vi "周期启动 (子VI).vi"   [LabVIEW 2016, in "质控单元.lvlib"]
types:
  T1 = cluster{"是否启用仪器":bool, "CODMn":cluster{"启动测量模式":cluster{"测量模式":enum16{"水样测量", "标样核查", "加标回收", "平行样", "校零", "校标"}}, "确定按钮":bool}, "启动模块":cluster{"氨氮":bool, "总磷":bool, "总氮":bool, "CODMn":bool, "CODCr":bool}, "常规启动":bool, "直接启动":bool}
  T2 = cluster{"周期设置类型":enum16{"定点启动", "间隔启动"}, "定时功能启用":bool, "定时间隔":dbl, "间隔启动次数 ":dbl, "已经启动次数 ":dbl, "24H周期设置":bool[], "模块选择":cluster{"氨氮":bool, "总磷":bool, "总氮":bool, "CODMn":bool, "CODCr":bool}, "采配水启用":bool}
  T3 = typedef "LVDateTimeRec.ctl" = cluster{"秒数的小数部分":dbl, "秒":i32, "分":i32, "时":i32, "日":i32, "月":i32, "年":i32, "天数（周）":i32, "天数（年）":i32, "DST":i32}
  T4 = cluster{"氨氮":bool, "总磷":bool, "总氮":bool, "CODMn":bool, "CODCr":bool}
  T5 = enum32{"Bad", "Idle", "Run top level", "Running"}
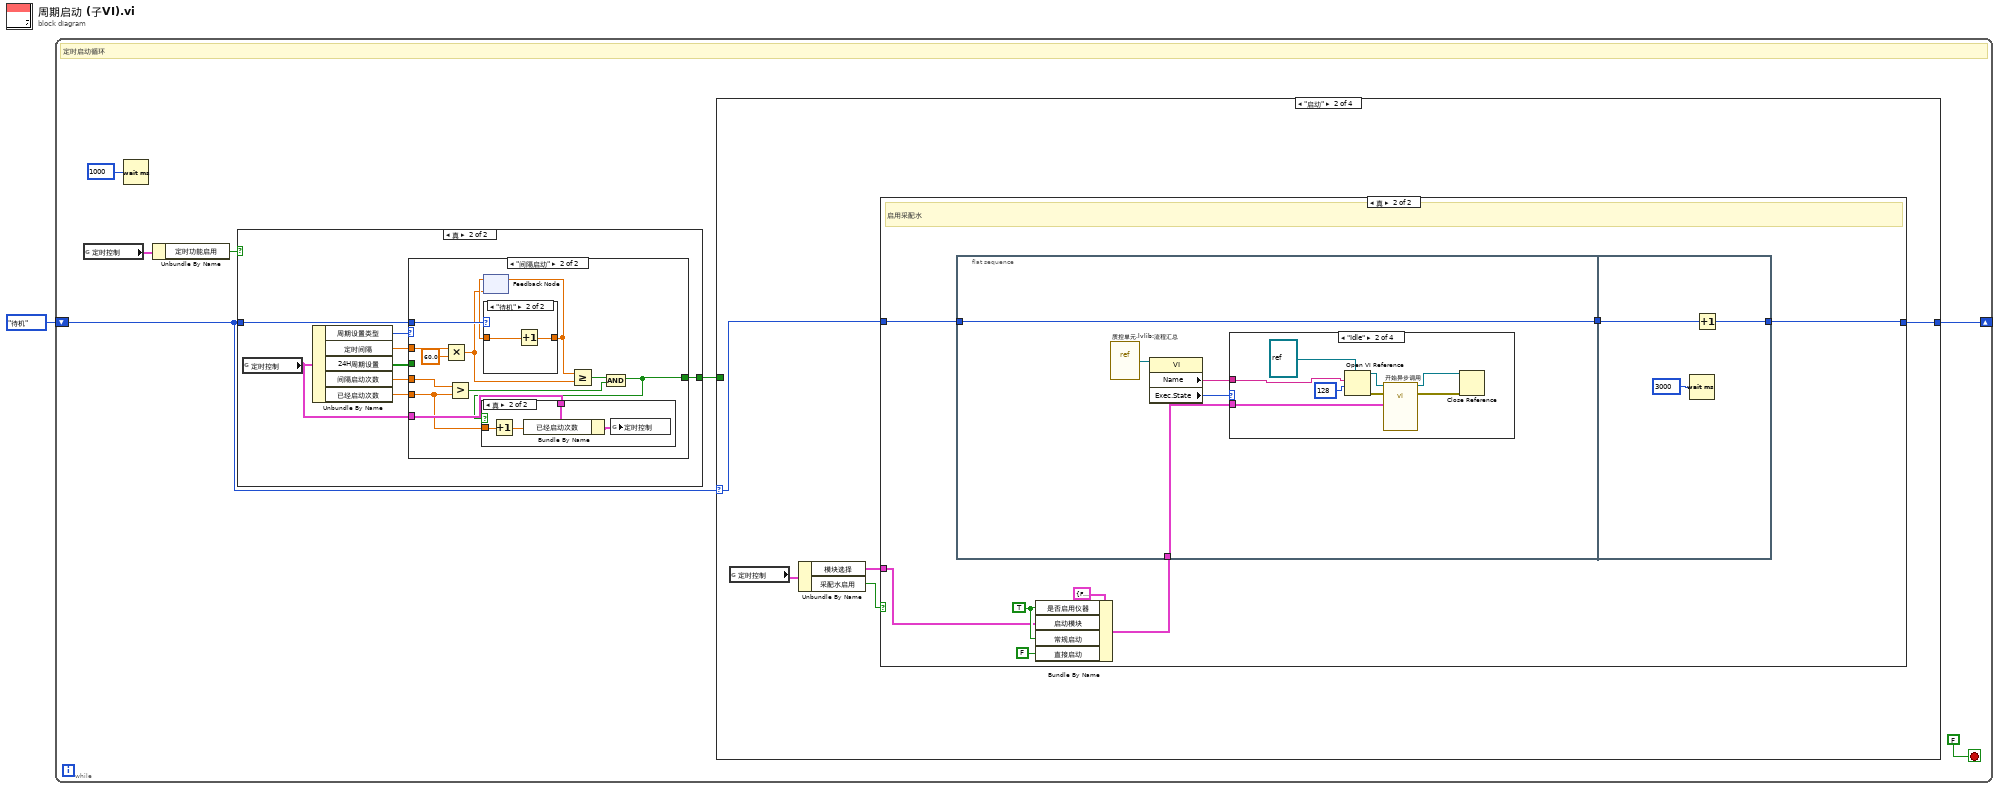
[diagram p0: block diagram]
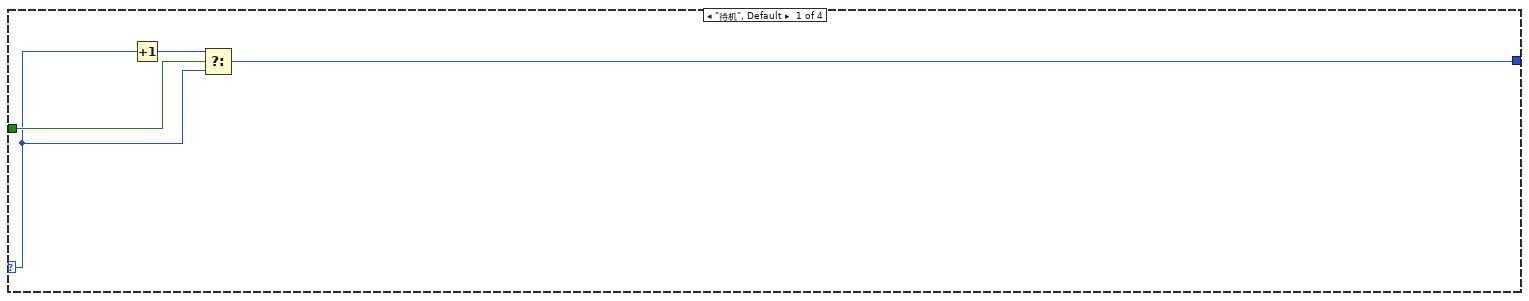
[diagram p2: hidden frame]
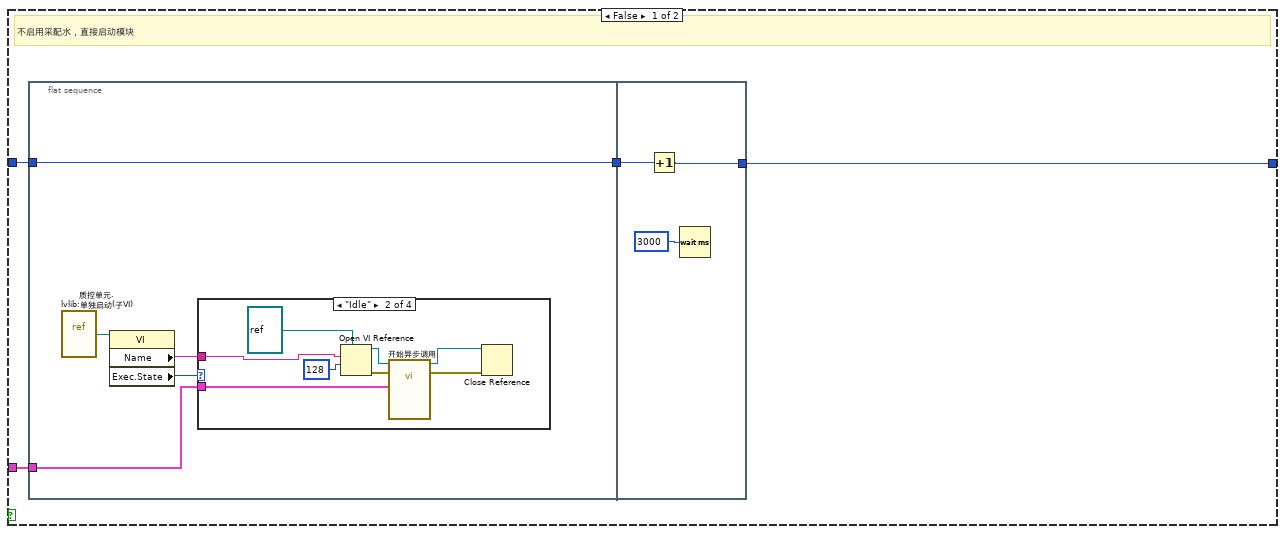
[diagram p3: hidden frame]
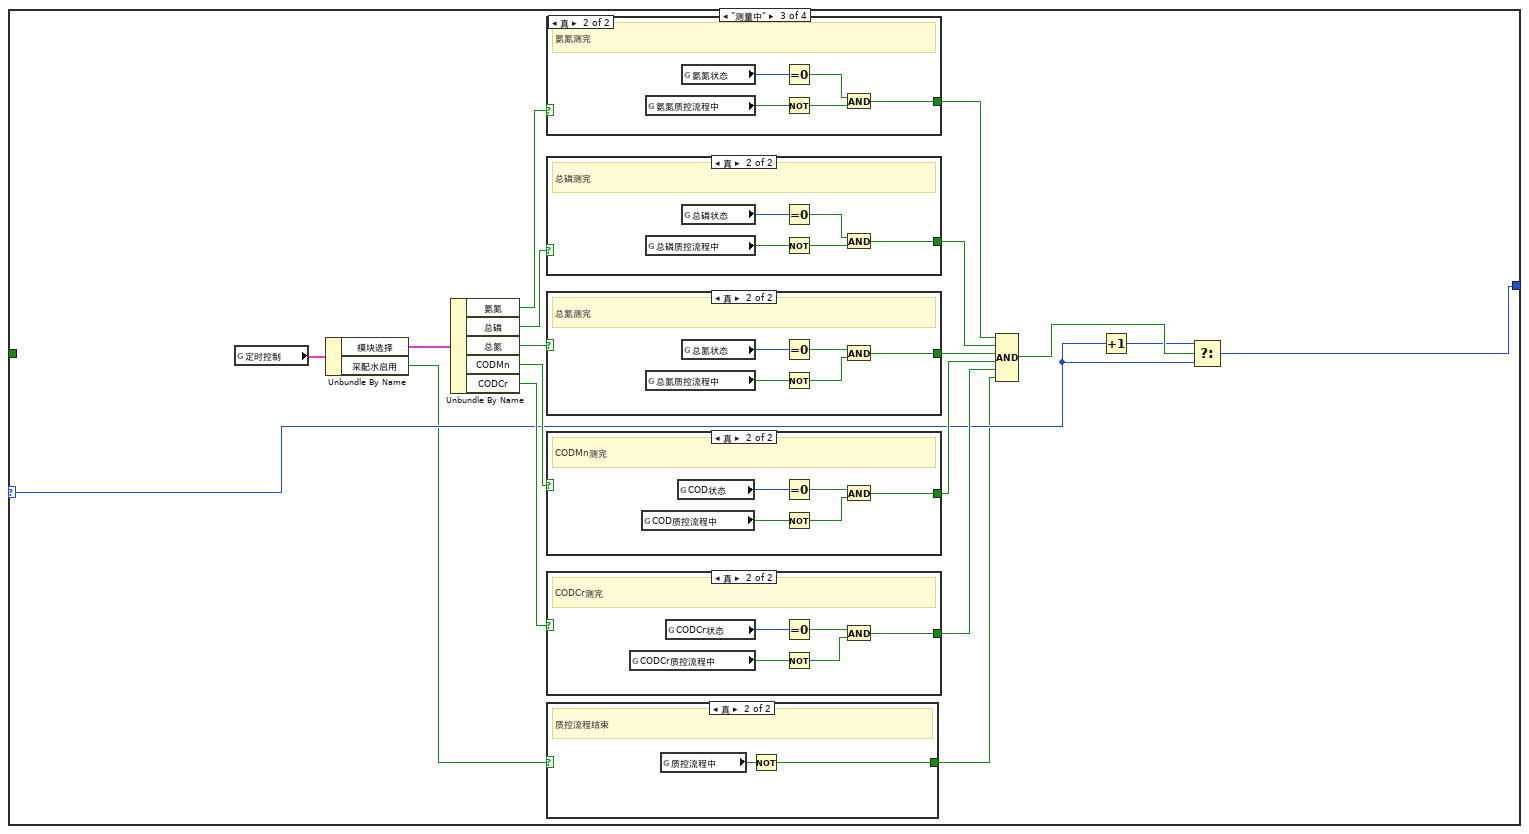
[diagram p10: hidden frame]
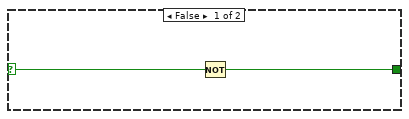
[diagram p11: hidden frame]
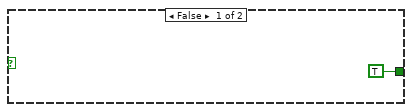
[diagram p12: hidden frame]
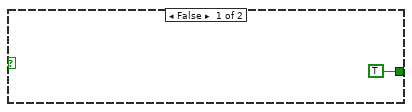
[diagram p13: hidden frame]
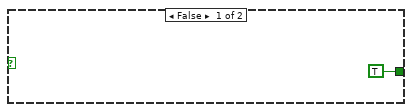
[diagram p14: hidden frame]
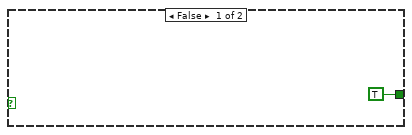
[diagram p15: hidden frame]
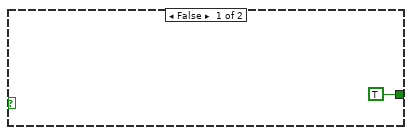
[diagram p16: hidden frame]
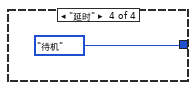
[diagram p17: hidden frame]
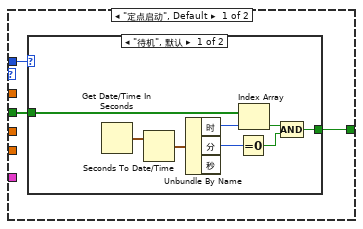
[diagram p19: hidden frame]
diagram:
  n1 = while {
    shift-right: [w6] -> _
    shift-left: enum16{"待机", "启动", "测量中", "延时"}."待机" -> [w5]
    stop <- FALSE stop-if-true
    # "定时启动循环"
    n2 = global read "断电保存全局.vi" "定时控制"() -> (w3:T2)
    n3 = Wait (ms)(milliseconds to wait=u32 1000 ("等待时间（毫秒）")) -> ()  [unwired: 1 out]
    n4 = Unbundle By Name(w3) -> ("定时功能启用"=w2:bool)
    n5 = case shown="真" w2 {
      tunnel: w5 -> [_ w119]
      tunnel: [_ w118] -> w4
      frame False {
      }
      frame True {
        n6 = global read "断电保存全局.vi" "定时控制"() -> (w115:T2)
        n7 = Unbundle By Name(w115) -> ("周期设置类型"=w120:enum16{"定点启动", "间隔启动"}, "定时间隔"=w121:dbl, "24H周期设置"=w122:bool[], "间隔启动次数"=w117:dbl, "已经启动次数"=w116:dbl)
        n8 = case shown="\"间隔启动\"" w120 {
          tunnel: w121 -> [_ w142]
          tunnel: w122 -> [w125 _]
          tunnel: w119 -> [w123 w145]
          tunnel: [w124 w134] -> w118
          tunnel: w117 -> [_ w138]
          tunnel: w116 -> [_ w135]
          tunnel: w115 -> [_ w136]
          frame "定点启动", Default {
            n9 = case shown="\"待机\", 默认" w123 {
              tunnel: w125 -> [w131 _]
              tunnel: [w126 _] -> w124
              frame "待机", Default {
                n10 = Get Date/Time In Seconds() -> (seconds since 1Jan1904=w133:timestamp)
                n11 = Seconds To Date/Time(time stamp (now)=w133) -> (date time rec=w132:T3)  [unwired: 1 in]
                n12 = Unbundle By Name(w132) -> ("时"=w130:i32, "分"=w129:i32)  [unwired: 1 out]
                n13 = Equal To 0?(x=w129) -> (x = 0?=w127:bool)
                n14 = Index Array(array=w131, index=w130) -> (element=w128:bool)
                n15 = Compound Arithmetic op=AND ("复合运算")(w128, w127) -> (w126:bool)
              }
              frame "启动" {
              }
            }
          }
          frame "间隔启动" {
            n16 = Multiply(x=w142, y=60.0) -> (x*y=w139:dbl)
            n17 = Greater?(x=w138, y=w135) -> (0:w137:bool)
            n18 = feedback #1(w139) -> (w144:dbl)
            n19 = case shown="\"待机\"" w145 {
              tunnel: w144 -> [_ w151]
              tunnel: [_ w150] -> w143
              frame Default {
              }
              frame "待机" {
                n20 = Increment(x=w151) -> (x+1=w150:dbl)
              }
            }
            n21 = feedback-in #1(w143) -> ()
            n22 = Greater Or Equal?(x=w143, y=w139) -> (x >= y?=w140:bool)
            n23 = And(x=w140, y=w137) -> (x .and. y?=w134:bool)
            n24 = case shown="真" w134 {
              tunnel: w136 -> [_ w149]
              tunnel: w135 -> [_ w148]
              frame False {
              }
              frame True {
                n25 = Increment(x=w148) -> (x+1=w147:dbl)
                n26 = Bundle By Name(cluster=w149, "已经启动次数"=w147) -> (w146:T2)
                n27 = global write "断电保存全局.vi" "定时控制"(w146) -> ()
              }
            }
          }
        }
      }
    }
    n28 = case shown="\"启动\"" w5 {
      selector: w5 -> [w9 w14 w65 _]
      tunnel: [w11 w17 w66 enum16{"待机", "启动", "测量中", "延时"}."待机"] -> w6
      tunnel: w4 -> [w12 _ _ _]
      frame "待机", Default {
        n29 = Increment(x=w9) -> (x+1=w10:enum16{"待机", "启动", "测量中", "延时"})
        n30 = Select(t=w10, s=w12, f=w9) -> (s? t:f=w11:enum16{"待机", "启动", "测量中", "延时"})
      }
      frame "启动" {
        n31 = global read "断电保存全局.vi" "定时控制"() -> (w15:T2)
        n32 = Unbundle By Name(w15) -> ("模块选择"=w16:T4, "采配水启用"=w13:bool)
        n33 = case shown="真" w13 {
          tunnel: [w20 w43] -> w17
          tunnel: w16 -> [w19 w39]
          tunnel: w14 -> [w18 w44]
          frame False {
            # "不启用采配水，直接启动模块"
            n34 = flat-sequence {
              tunnel: w19 -> [w22]
              tunnel: w18 -> [w26]
              tunnel: [w26] -> w21
              tunnel: [w37] -> w20
              tunnel: w21 -> [w36]
              frame #0 {
                n35 = vi-ref "质控单元.lvlib:单独启动(子VI).vi"() -> (w24:refnum<vi>)
                n36 = property class="VI"(reference=w24) -> ("Name"=w25:string, "Exec.State"=w23:T5)  [unwired: 1 in, 2 out]
                n37 = case shown="\"Idle\"" w23 {
                  tunnel: w25 -> [_ w33 _ _]
                  tunnel: w22 -> [_ w27 _ _]
                  frame "Bad", Default {
                  }
                  frame "Idle" {
                    n38 = Open VI Reference(type specifier VI Refnum (for type only)=refnum<vi> refnum ("类型说明符VI引用句柄（仅用于类型）"), vi path=w33, options=128 ("选项")) -> (vi reference=w34:refnum<vi>, error out=w30:errorcluster)  [unwired: 3 in]
                    n39 = call-by-ref "开始异步调用"(reference=w34, error in=w30, "启动模块"=w27) -> (reference out=w32:refnum<vi>, error out=w31:errorcluster)  [unwired: 11 in]
                    n40 = Close Reference(reference=w32, error in (no error)=w31) -> ()  [unwired: 1 out]
                  }
                  frame "Run top level" {
                  }
                  frame "Running" {
                  }
                }
              }
              frame #1 {
                n41 = Increment(x=w36) -> (x+1=w37:enum16{"待机", "启动", "测量中", "延时"})
                n42 = Wait (ms)(milliseconds to wait=u32 3000 ("等待时间（毫秒）")) -> ()  [unwired: 1 out]
              }
            }
          }
          frame True {
            w41 = TRUE ("是否启用仪器")
            # "启用采配水"
            n43 = flat-sequence {
              tunnel: [w50] -> w45
              tunnel: w44 -> [w50]
              tunnel: w38 -> [w46]
              tunnel: w45 -> [w61]
              tunnel: [w60] -> w43
              frame #0 {
                n44 = vi-ref "质控单元.lvlib:流程汇总.vi"() -> (w48:refnum<vi>)
                n45 = property class="VI"(reference=w48) -> ("Name"=w49:string, "Exec.State"=w47:T5)  [unwired: 1 in, 2 out]
                n46 = case shown="\"Idle\"" w47 {
                  tunnel: w49 -> [_ w57 _ _]
                  tunnel: w46 -> [_ w51 _ _]
                  frame "Bad", Default {
                  }
                  frame "Idle" {
                    n47 = Open VI Reference(type specifier VI Refnum (for type only)=refnum<vi> refnum ("类型说明符VI引用句柄（仅用于类型）"), vi path=w57, options=128 ("选项")) -> (vi reference=w58:refnum<vi>, error out=w54:errorcluster)  [unwired: 3 in]
                    n48 = call-by-ref "开始异步调用"(reference=w58, error in=w54, "参数"=w51) -> (reference out=w56:refnum<vi>, error out=w55:errorcluster)  [unwired: 11 in]
                    n49 = Close Reference(reference=w56, error in (no error)=w55) -> ()  [unwired: 1 out]
                  }
                  frame "Run top level" {
                  }
                  frame "Running" {
                  }
                }
              }
              frame #1 {
                n50 = Wait (ms)(milliseconds to wait=u32 3000 ("等待时间（毫秒）")) -> ()  [unwired: 1 out]
                n51 = Increment(x=w61) -> (x+1=w60:enum16{"待机", "启动", "测量中", "延时"})
              }
            }
            n52 = Bundle By Name(cluster=T1 {"是否启用仪器"=FALSE, "CODMn"={"启动测量模式"={"测量模式"=enum."水样测量"}, "确定按钮"=FALSE}, "启动模块"={"氨氮"=FALSE, "总磷"=FALSE, "总氮"=FALSE, "CODMn"=FALSE, "CODCr"=FALSE}, "常规启动"=FALSE, "直接启动"=FALSE} ("参数"), "是否启用仪器"=w41, "启动模块"=w39, "常规启动"=w41, "直接启动"=FALSE) -> (w38:T1)
          }
        }
      }
      frame "测量中" {
        n53 = global read "断电保存全局.vi" "定时控制"() -> (w79:T2)
        n54 = Unbundle By Name(w79) -> ("模块选择"=w78:T4, "采配水启用"=w64:bool)
        n55 = Unbundle By Name(w78) -> ("氨氮"=w71:bool, "总磷"=w70:bool, "总氮"=w69:bool, "CODMn"=w68:bool, "CODCr"=w67:bool)
        n56 = case shown="真" w71 {
          tunnel: [TRUE w111] -> w72
          frame False {
          }
          frame True {
            # "氨氮测完"
            n57 = global read "质控测完标志全局 1.vi" "氨氮质控流程中"() -> (w113:bool)
            n58 = global read "加标回收状态全局变量.vi" "氨氮状态"() -> (w110:u16)
            n59 = Equal To 0?(x=w110) -> (x = 0?=w109:bool)
            n60 = Not(x=w113) -> (.not. x?=w112:bool)
            n61 = And(x=w109, y=w112) -> (x .and. y?=w111:bool)
          }
        }
        n62 = case shown="真" w70 {
          tunnel: [TRUE w105] -> w73
          frame False {
          }
          frame True {
            # "总磷测完"
            n63 = global read "质控测完标志全局 1.vi" "总磷质控流程中"() -> (w107:bool)
            n64 = global read "加标回收状态全局变量.vi" "总磷状态"() -> (w104:u16)
            n65 = Equal To 0?(x=w104) -> (x = 0?=w103:bool)
            n66 = Not(x=w107) -> (.not. x?=w106:bool)
            n67 = And(x=w103, y=w106) -> (x .and. y?=w105:bool)
          }
        }
        n68 = case shown="真" w69 {
          tunnel: [TRUE w99] -> w74
          frame False {
          }
          frame True {
            # "总氮测完"
            n69 = global read "质控测完标志全局 1.vi" "总氮质控流程中"() -> (w101:bool)
            n70 = global read "加标回收状态全局变量.vi" "总氮状态"() -> (w98:u16)
            n71 = Equal To 0?(x=w98) -> (x = 0?=w97:bool)
            n72 = Not(x=w101) -> (.not. x?=w100:bool)
            n73 = And(x=w97, y=w100) -> (x .and. y?=w99:bool)
          }
        }
        n74 = case shown="真" w68 {
          tunnel: [TRUE w93] -> w75
          frame False {
          }
          frame True {
            # "CODMn测完"
            n75 = global read "质控测完标志全局 1.vi" "COD质控流程中"() -> (w95:bool)
            n76 = global read "加标回收状态全局变量.vi" "COD状态"() -> (w92:u16)
            n77 = Equal To 0?(x=w92) -> (x = 0?=w91:bool)
            n78 = Not(x=w95) -> (.not. x?=w94:bool)
            n79 = And(x=w91, y=w94) -> (x .and. y?=w93:bool)
          }
        }
        n80 = case shown="真" w67 {
          tunnel: [TRUE w87] -> w76
          frame False {
          }
          frame True {
            # "CODCr测完"
            n81 = global read "质控测完标志全局 1.vi" "CODCr质控流程中"() -> (w89:bool)
            n82 = global read "加标回收状态全局变量.vi" "CODCr状态"() -> (w86:u16)
            n83 = Equal To 0?(x=w86) -> (x = 0?=w85:bool)
            n84 = Not(x=w89) -> (.not. x?=w88:bool)
            n85 = And(x=w85, y=w88) -> (x .and. y?=w87:bool)
          }
        }
        n86 = case shown="真" w64 {
          selector: w64 -> [w81 _]
          tunnel: [w80 w82] -> w63
          frame False {
            n87 = Not(x=w81) -> (.not. x?=w80:bool)
          }
          frame True {
            # "质控流程结束"
            n88 = global read "质控测完标志全局 1.vi" "质控流程中"() -> (w83:bool)
            n89 = Not(x=w83) -> (.not. x?=w82:bool)
          }
        }
        n90 = Compound Arithmetic op=AND ("复合运算")(w72, w73, w74, w75, w76, w63) -> (w77:bool)
        n91 = Increment(x=w65) -> (x+1=w62:enum16{"待机", "启动", "测量中", "延时"})
        n92 = Select(t=w62, s=w77, f=w65) -> (s? t:f=w66:enum16{"待机", "启动", "测量中", "延时"})
      }
      frame "延时" {
      }
    }
  }
